vi "Bitwise XOR (Greyscale).vi"(8 "error in (no error)":errorcluster, 9 "Greyscale Image Destination in":T1, 10 "Greyscale Image B in":T1, 11 "Greyscale Image A in":T1) -> (0 "error out":errorcluster, 3 "Greyscale Image Destination":T1)   [LabVIEW 2020, in "image.lvlib"]
doc: "Compute the bitwise XOR of the pixels in the A and B input images."
uses:
  image.lvlib
  Greyscale Image.ctl
  BitwiseOperation.ctl
  253e84a8-32ce-4670-ae81-0d341c439dd3.vi
  <vilib>/Utility/error.llb/Error Cluster From Error Code.vi
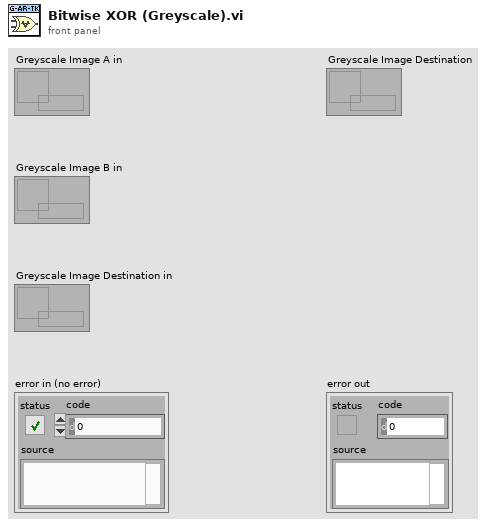
[diagram p1: front panel]
types:
  T1 = typedef "image.lvlib/Greyscale Image.ctl" = refnum<data-value>
  T2 = typedef "image.lvlib/BitwiseOperation.ctl" = enum8{"OR", "AND", "XOR"}
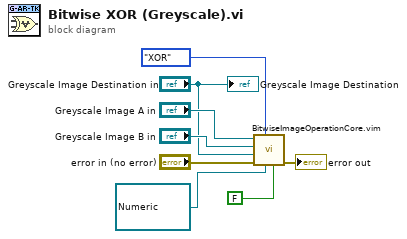
[diagram p0: block diagram]
diagram:
  n1 = call "BitwiseImageOperationCore.vim"("HasMask"=FALSE, "Mask"=refnum<data-value> refnum, "BitwiseOperation"=BitwiseOperation."XOR", "error in (no error)"="error in (no error)", "Destination Image"="Greyscale Image Destination in", "Image B"="Greyscale Image B in", "Image A"="Greyscale Image A in") -> ("error out"=→"error out":errorcluster)  [unwired: 4 in]
  "Greyscale Image Destination" <- "Greyscale Image Destination in"
